vi "GCS3_Rename_Units.vi"(0 "System No.":i32, 1 "Axes":string[](array[string]), 5 "error in (no error)":errorcluster, 7 "Target Unit":string) -> (14 "GCS 3.0 Units":string[](array[string]), 19 "error out":errorcluster)   [LabVIEW 2026]
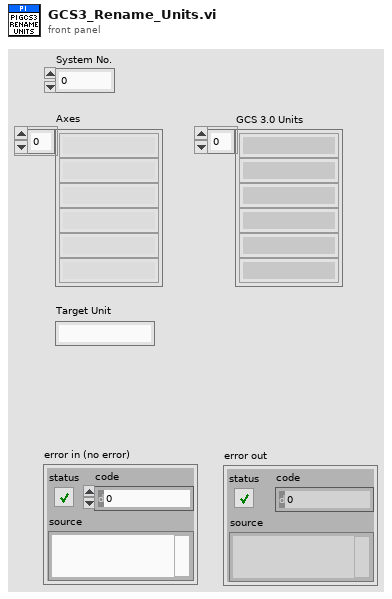
[diagram p1: front panel]
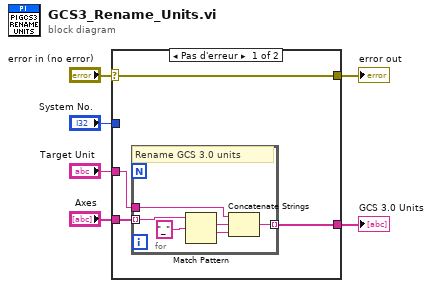
[diagram p0: block diagram]
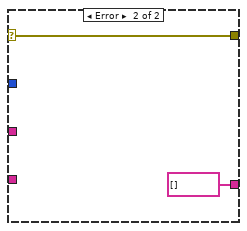
[diagram p2: hidden frame]
diagram:
  n1 = case shown="Pas d'erreur" "error in (no error)" {
    selector: "error in (no error)" -> [w10 w18]
    tunnel: [w10 w18] -> w5
    tunnel: "Target Unit" -> [w7 _]
    tunnel: "Axes" -> [w9 _]
    tunnel: "System No." -> [_ _]
    tunnel: [w8 string[] [] ("GCS 3.0 Units")] -> w1
    frame No Error {
      n2 = for {
        tunnel: w9 -> [w15] mode=indexing
        tunnel: [w11] -> w8 mode=indexing
        tunnel: w7 -> [w14]
        # "Rename GCS 3.0 units"
        n3 = Match Pattern(string=w15, regular expression="_") -> (match substring=w13:string, after substring=w12:string)  [unwired: 1 in, 2 out]
        n4 = Concatenate Strings(w14, w13, w12) -> (w11:string)
      }
    }
    frame Error {
    }
  }
  "error out" <- w5
  "GCS 3.0 Units" <- w1
